vi "Defender_din.vi"(9 "balls":T1[](array[typedef]), 10 "IA State":T2={"our_robots"=[], "enemy_robots"=[], "balls"=[], "geometry"={"field_length"=0, "field_width"=0, "goal_width"=0, "goal_depth"=0, "center_circle_radius"=0, "defense_width"=0, "defense_depth"=0, "free_kick_from_defense_dist"=0, "penalty_spot_from_field_line_dist"=0, "penalty_line_from_spot_dist"=0, "half_moon_depth"=0, "half_moon_width"=0}, "IA Judge"={"stage"="", "command"="", "our_goalie_id"=0.0, "enemy_goalie_id"=0.0, "command enum"=enum."Halt", "Time"=enum."Azul"}, "Received Timestamp"=timestamp(0 s since 1904-01-01), "Events"={"Touch"=FALSE, "id touch"=0.0, "Ball out of \nVision"=FALSE, "Ball inside \nGoalie area"=FALSE, "Robot not responding"=FALSE, "Robots responding status"=[1.0, 1.0, 1.0, 1.0, 1.0, 1.0], "Enemy Ball \nPossession"=FALSE, "Id ini Possession"=0.0, "Ball Possesion"=FALSE, "Id Possesion"=0.0, "Ball at\nour goal side"=FALSE, "Ball at\ntouchline"=FALSE, "Ball at\nenemy goal side"=FALSE}}, 11 "Robot in":T3) -> (3 "Robot out":T3)   [LabVIEW 2018]
uses:
  Core/AI Robot.ctl
  Functions Enum.ctl
  AttackerStates.ctl
  Path Planning/RRT/PathDests.ctl
  Path Planning/RRT/PathDest.ctl
  Core/AI Input.ctl
  Core/AI Ball.ctl
  Core/Field Size.ctl
  Core/AI Judge.ctl
  Command Enum.ctl
  Util/Events/Events.ctl
  <vilib>/Analysis/_algsub.llb/Real Vector Norm.vi
  <vilib>/Analysis/NI_AALPro.lvlib
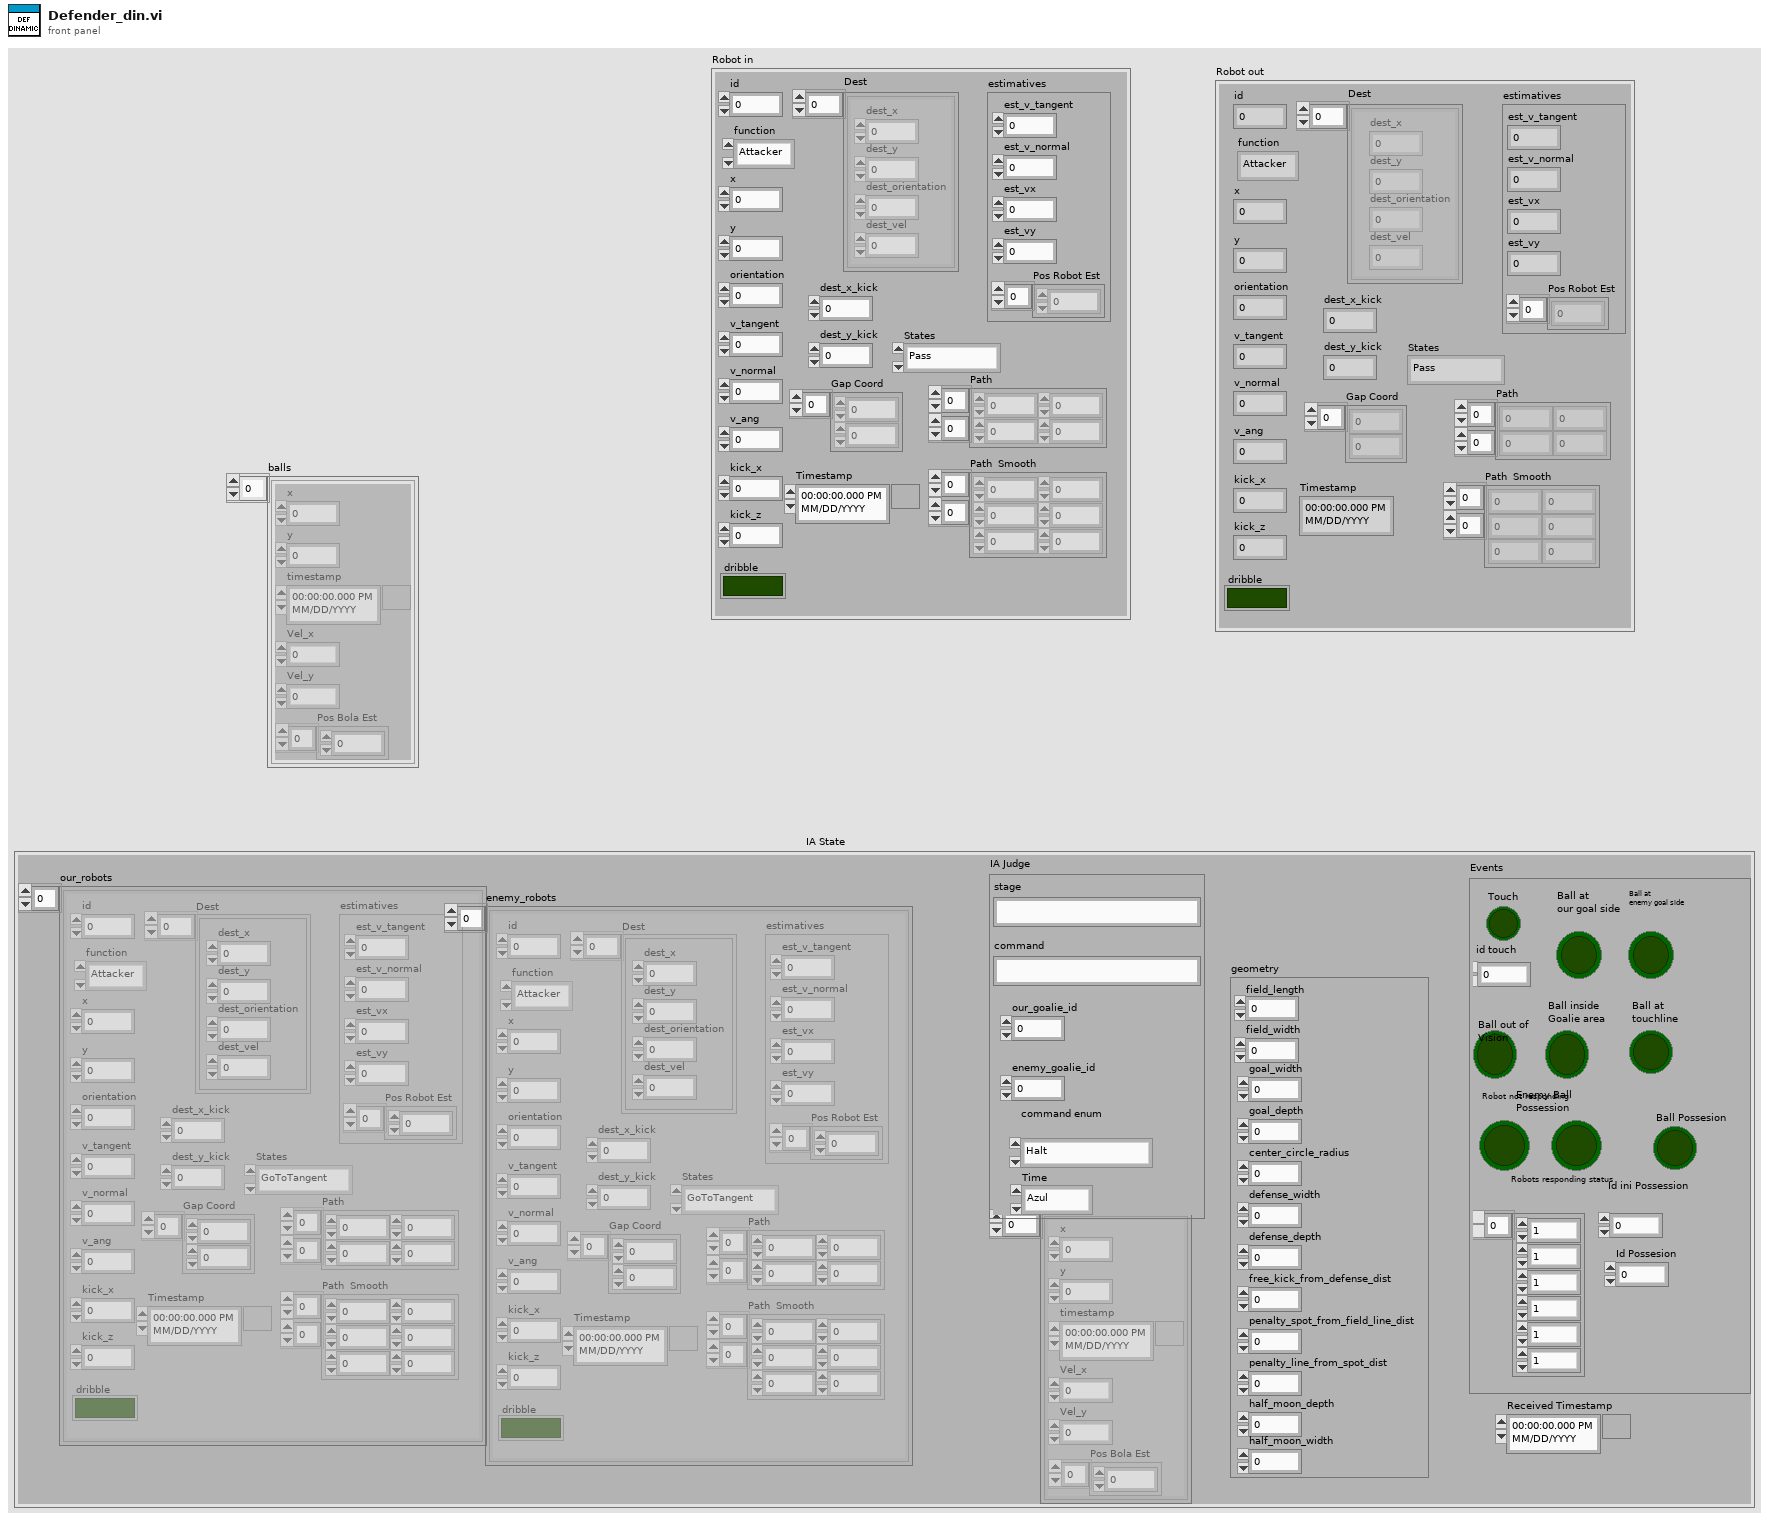
[diagram p1: front panel]
types:
  T1 = typedef "AI Ball.ctl" = cluster{"x":dbl, "y":dbl, "timestamp":timestamp, "Vel_x":dbl, "Vel_y":dbl, "Pos Bola Est":dbl[]}
  T2 = typedef "AI Input.ctl" = cluster{"our_robots":T3[], "enemy_robots":T3[], "balls":T1[], "geometry":T8, "IA Judge":T9, "Received Timestamp":timestamp, "Events":T11}
  T3 = typedef "AI Robot.ctl" = cluster{"id":u32, "function":T4, "x":dbl, "y":dbl, "orientation":dbl, "v_tangent":dbl, "v_normal":dbl, "v_ang":dbl, "kick_x":dbl, "kick_z":dbl, "dribble":bool, "Timestamp":timestamp, "estimatives":cluster{"est_v_tangent":dbl, "est_v_normal":dbl, "est_vx":dbl, "est_vy":dbl, "Pos Robot Est":dbl[]}, "dest_x_kick":dbl, "dest_y_kick":dbl, "Gap Coord":dbl[], "States":T5, "Path ":dbl[][], "Path  Smooth":dbl[][], "Dest":T6}
  T4 = typedef "Functions Enum.ctl" = enum16{"Attacker", "Goalie", "Defender", "Striker", "Goto 0", "Dummy", "Kicker", "ZigZag"}
  T5 = typedef "AttackerStates.ctl" = enum16{"Pass", "GoToTangent", "BallGetting", "GoToKick", "Rotate anti-clockwise", "Rotate Clockwise", ""}
  T6 = typedef "PathDests.ctl" = T7[]
  T7 = typedef "PathDest.ctl" = cluster{"dest_x":dbl, "dest_y":dbl, "dest_orientation":dbl, "dest_vel":dbl}
  T8 = typedef "Field Size.ctl" = cluster{"field_length":u32, "field_width":u32, "goal_width":u32, "goal_depth":u32, "center_circle_radius":u32, "defense_width":u32, "defense_depth":u32, "free_kick_from_defense_dist":u32, "penalty_spot_from_field_line_dist":u32, "penalty_line_from_spot_dist":u32, "half_moon_depth":u32, "half_moon_width":u32}
  T9 = typedef "AI Judge.ctl" = cluster{"stage":string, "command":string, "our_goalie_id":dbl, "enemy_goalie_id":dbl, "command enum":T10, "Time":enum16{"Azul", "Amarelo"}}
  T10 = typedef "Command Enum.ctl" = enum16{"Halt", "Stop", "Force Start", "PKA Normal Start", "Prepare Kickoff Ally", "PKE Normal Start", "Prepare Kickoff Enemy", "Prepare Penalty Ally", "PPA Normal Start", "Prepare Penalty Enemy", "PPE Normal Start", "Ball Placement Enemy Up", "Ball Placement Enemy Down", "Ball Placement Ally Up", "Ball Placement Ally Mid", "Ball Placement Ally Down", "Indirect Free Enemy", "Indirect Free Ally", "Timeout Enemy", "Timeout Ally", "Goal Enemy", "Goal Ally", "Normal Half Time", "Extra Time Break", "Extra Half Time", "None", "Post Game"}
  T11 = typedef "Events.ctl" = cluster{"Touch":bool, "id touch":dbl, "Ball out of \nVision":bool, "Ball inside \nGoalie area":bool, "Robot not responding":bool, "Robots responding status":dbl[], "Enemy Ball \nPossession":bool, "Id ini Possession":dbl, "Ball Possesion":bool, "Id Possesion":dbl, "Ball at\nour goal side":bool, "Ball at\ntouchline":bool, "Ball at\nenemy goal side":bool}
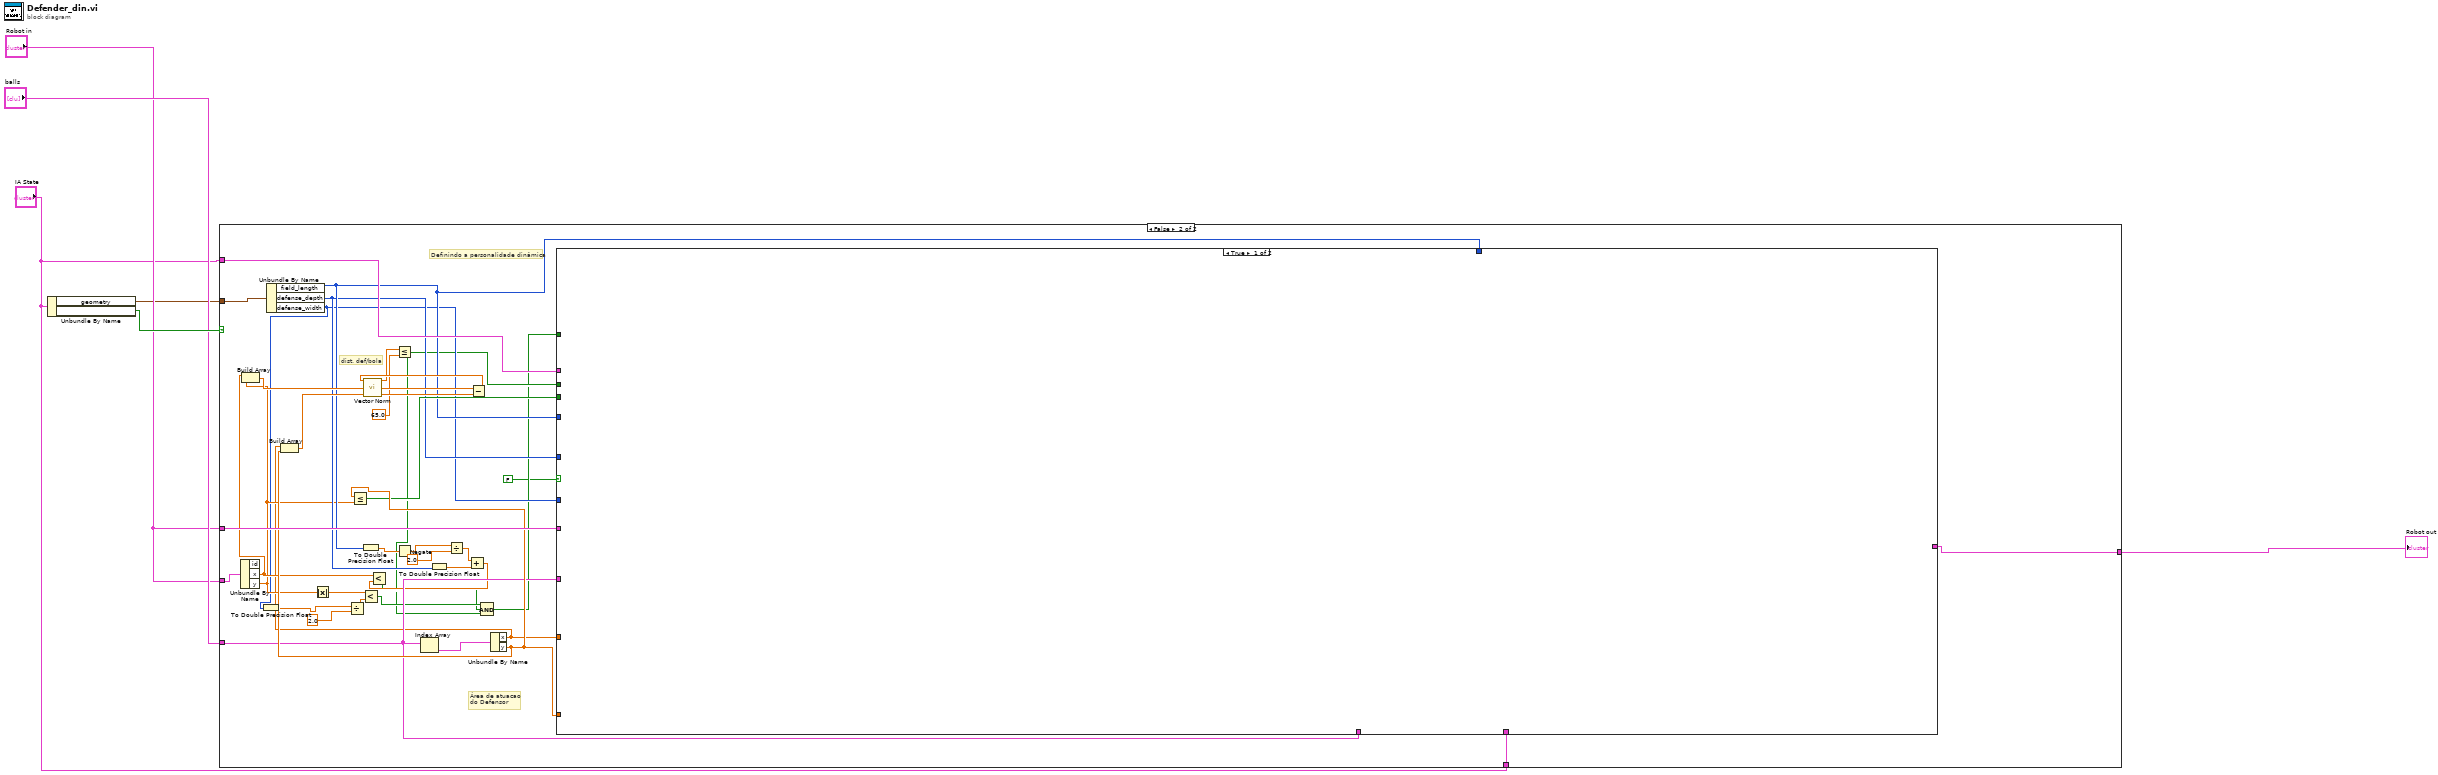
[diagram p0: block diagram]
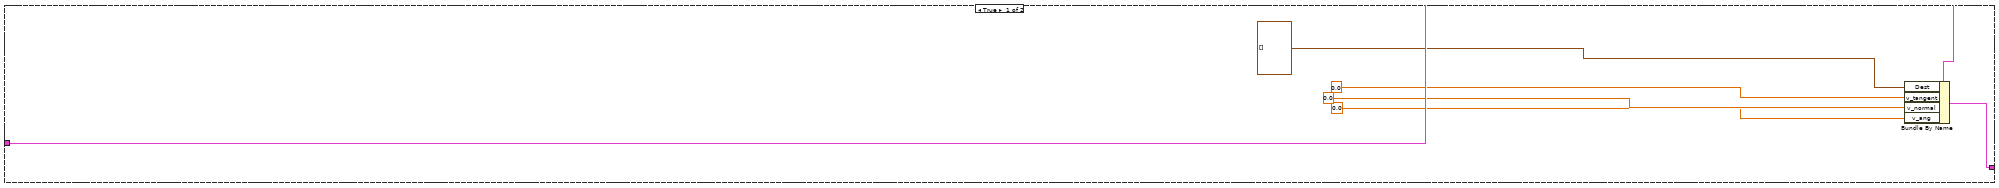
[diagram p2: hidden frame]
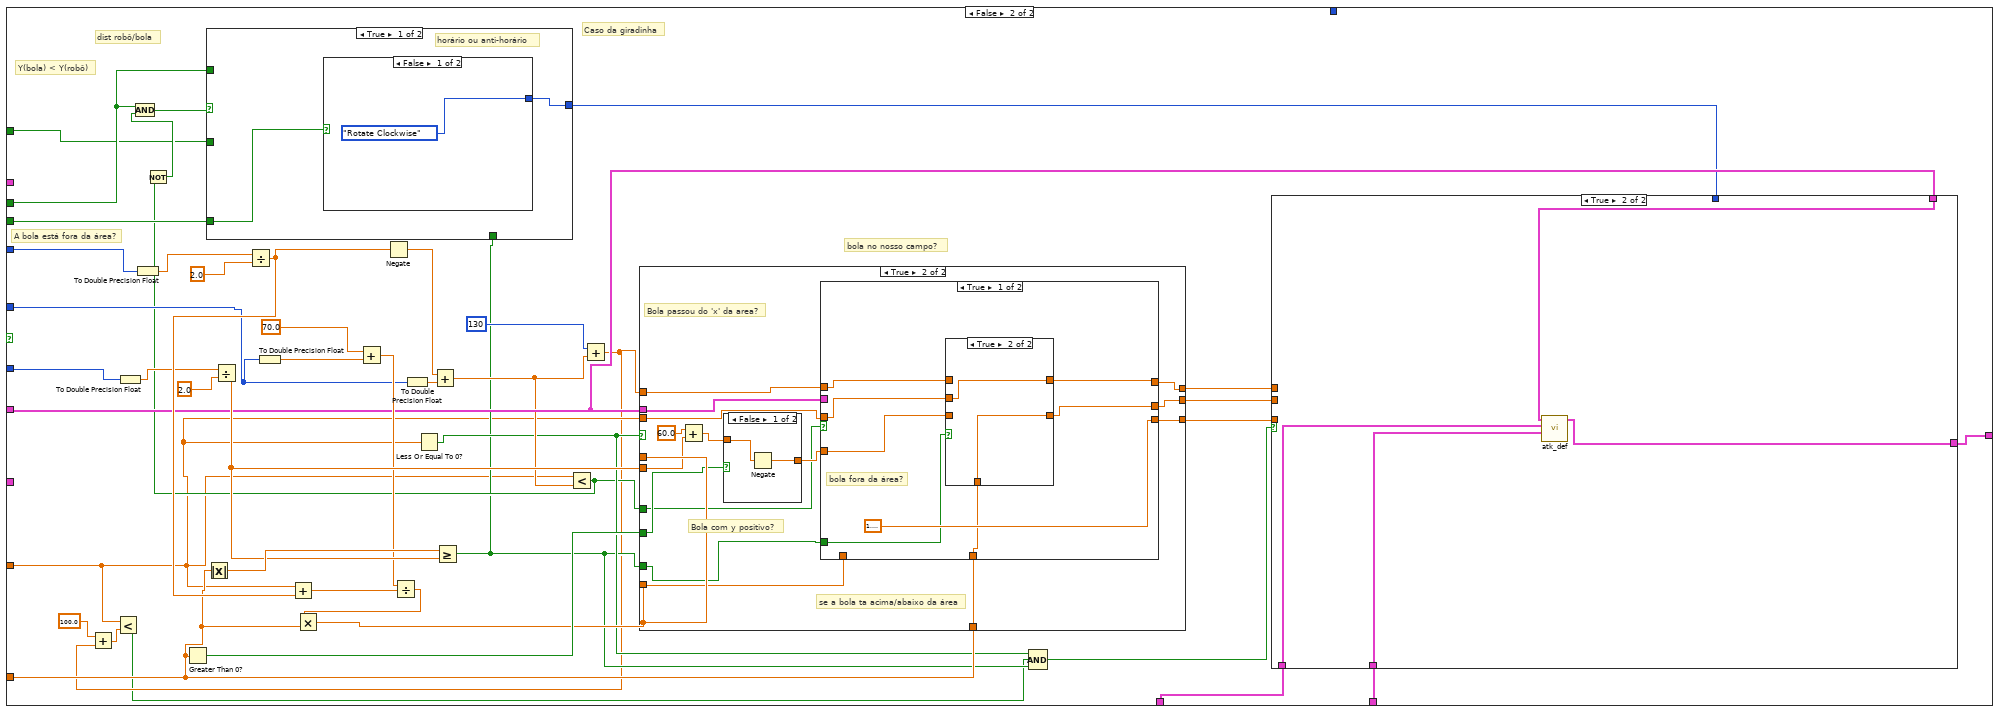
[diagram p3: hidden frame]
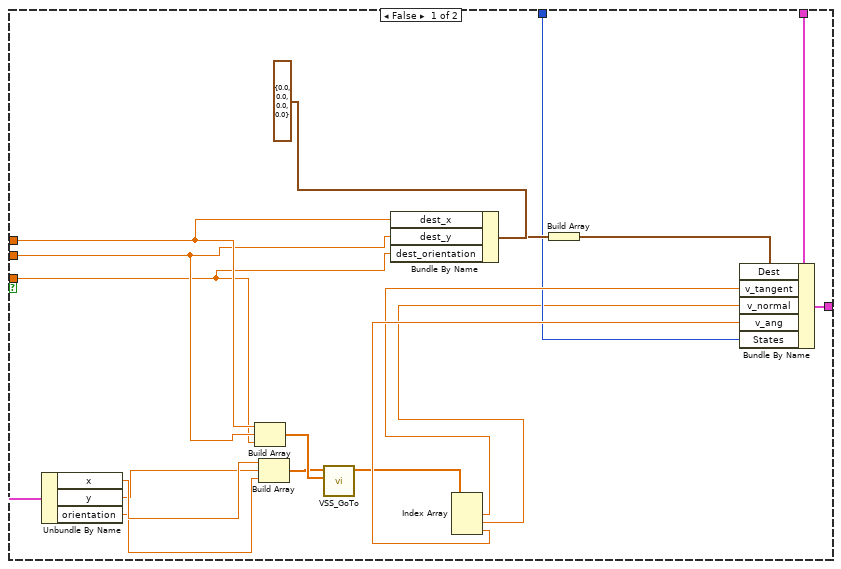
[diagram p4: hidden frame]
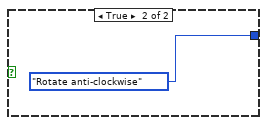
[diagram p5: hidden frame]
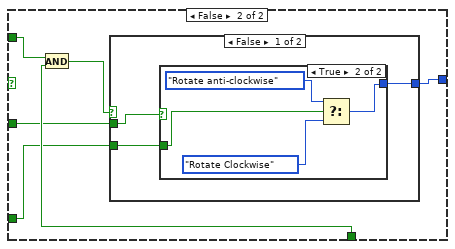
[diagram p6: hidden frame]
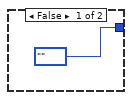
[diagram p7: hidden frame]
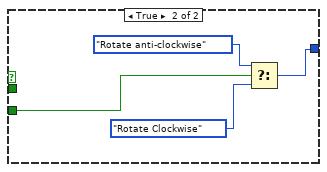
[diagram p8: hidden frame]
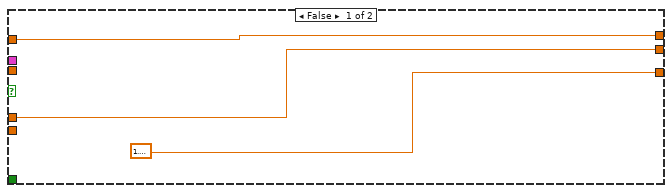
[diagram p9: hidden frame]
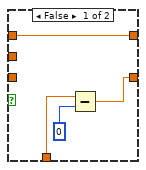
[diagram p11: hidden frame]
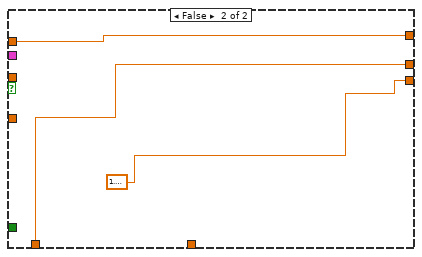
[diagram p12: hidden frame]
diagram:
  n1 = Unbundle By Name("IA State") -> ("geometry"=w3:T8, "Events.Ball out of \nVision"=w6:bool)
  n2 = case shown="False" w6 {
    tunnel: "Robot in" -> [w11 w48]
    tunnel: "balls" -> [_ w35]
    tunnel: "Robot in" -> [_ w46]
    tunnel: w3 -> [_ w45]
    tunnel: "IA State" -> [_ w44]
    tunnel: [w12 w43] -> w2
    tunnel: "IA State" -> [_ w34]
    frame True {
      n3 = Bundle By Name(cluster=w11, "Dest"=T7[] [], "v_tangent"=0.0, "v_normal"=0.0, "v_ang"=0.0) -> (w12:T3)
    }
    frame False {
      # "Área de atuacao\ndo Defensor"
      # "dist. def/bola"
      # "Definindo a personalidade dinâmica"
      n4 = Unbundle By Name(w46) -> ("x"=w33:dbl, "y"=w24:dbl)  [unwired: 1 out]
      n5 = Build Array(w33, w24) -> (w42:dbl[])
      n6 = Unbundle By Name(w45) -> ("field_length"=w29:u32, "defense_depth"=w27:u32, "defense_width"=w21:u32)
      n7 = To Double Precision Float(number=w21) -> (double precision float=w15:dbl)
      n8 = Absolute Value(x=w24) -> (abs(x)=w23:dbl)
      n9 = Divide(x=w15, y=2.0) -> (x/y=w20:dbl)
      n10 = To Double Precision Float(number=w29) -> (double precision float=w30:dbl)
      n11 = Less?(x=w23, y=w20) -> (x < y?=w19:bool)
      n12 = Negate(x=w30) -> (-x=w31:dbl)
      n13 = Index Array(array=w35) -> (element=w47:T1)  [unwired: 1 in]
      n14 = To Double Precision Float(number=w27) -> (double precision float=w26:dbl)
      n15 = Divide(x=w31, y=2.0) -> (x/y=w28:dbl)
      n16 = Add(x=w28, y=w26) -> (x+y=w25:dbl)
      n17 = Less?(x=w33, y=w25) -> (x < y?=w18:bool)
      n18 = Unbundle By Name(w47) -> ("x"=w14:dbl, "y"=w37:dbl)
      n19 = Build Array(w14, w37) -> (w41:dbl[])
      n20 = Less Or Equal?(x=w37, y=w24) -> (x <= y?=w36:bool)
      n21 = Subtract(x=w42, y=w41) -> (x-y=w40:dbl[])
      n22 = call-poly <vilib>:"Vector Norm.vi"("Input Vector"=w40) -> ("norm"=w39:dbl)  [unwired: 9 in, 1 out]
      n23 = Less Or Equal?(x=w39, y=65.0) -> (x <= y?=w17:bool)
      n24 = Compound Arithmetic op=AND(w19, w18, w17) -> (w16:bool)
      n25 = case shown="True" FALSE {
        tunnel: w48 -> [_ w75]
        tunnel: w14 -> [_ w53]
        tunnel: w37 -> [_ w79]
        tunnel: w29 -> [_ w73]
        tunnel: w27 -> [_ w70]
        tunnel: w21 -> [_ w67]
        tunnel: w44 -> [_ _]
        tunnel: w35 -> [_ _]
        tunnel: [_ w74] -> w43
        tunnel: w17 -> [_ w61]
        tunnel: w36 -> [_ w64]
        tunnel: w35 -> [_ w56]
        tunnel: w29 -> [_ _]
        tunnel: w34 -> [_ w55]
        tunnel: w16 -> [_ w54]
        frame True {
        }
        frame False {
          # "Y(bola) < Y(robô)"
          # "dist robô/bola"
          # "A bola está fora da área?"
          # "Caso da giradinha"
          # "bola no nosso campo?"
          n26 = To Double Precision Float(number=w67) -> (double precision float=w66:dbl)
          n27 = To Double Precision Float(number=w73) -> (double precision float=w72:dbl)
          n28 = Greater Than 0?(x=w79) -> (x > 0?=w86:bool)
          n29 = Absolute Value(x=w79) -> (abs(x)=w91:dbl)
          n30 = Divide(x=w66, y=2.0) -> (x/y=w83:dbl)
          n31 = Divide(x=w72, y=2.0) -> (x/y=w85:dbl)
          n32 = To Double Precision Float(number=w70) -> (double precision float=w71:dbl)
          n33 = Add(x=w53, y=w85) -> (x+y=w84:dbl)
          n34 = Add(x=70.0, y=w71) -> (x+y=w81:dbl)
          n35 = Negate(x=w85) -> (-x=w90:dbl)
          n36 = Divide(x=w81, y=w84) -> (x/y=w88:dbl)
          n37 = Multiply(x=w88, y=w79) -> (x*y=w80:dbl)
          n38 = To Double Precision Float(number=w70) -> (double precision float=w69:dbl)
          n39 = Less Or Equal To 0?(x=w53) -> (x <= 0?=w60:bool)
          n40 = Add(x=w90, y=w69) -> (x+y=w62:dbl)
          n41 = Greater Or Equal?(x=w91, y=w83) -> (x >= y?=w58:bool)
          n42 = Less?(x=w53, y=w62) -> (x < y?=w59:bool)
          n43 = Not(x=w59) -> (.not. x?=w63:bool)
          n44 = Compound Arithmetic op=AND(w61, w63) -> (w65:bool)
          n45 = case shown="True" w65 {
            tunnel: [w115 w124] -> w68
            tunnel: w64 -> [w116 w120]
            tunnel: w61 -> [_ w123]
            tunnel: w58 -> [_ w122]
            tunnel: w54 -> [_ w119]
            frame True {
              # "horário ou anti-horário"
              n46 = case shown="False" w116 {
                tunnel: [AttackerStates."Rotate Clockwise" ("States") AttackerStates."Rotate anti-clockwise" ("States")] -> w115
                frame False {
                }
                frame True {
                }
              }
            }
            frame False {
              n47 = And(x=w123, y=w122) -> (x .and. y?=w121:bool)
              n48 = case shown="False" w121 {
                tunnel: [w127 w135] -> w124
                tunnel: w120 -> [w125 w136]
                tunnel: w119 -> [w126 _]
                frame False {
                  n49 = case shown="True" w126 {
                    tunnel: [AttackerStates."" ("States") w129] -> w127
                    tunnel: w125 -> [_ w130]
                    frame False {
                    }
                    frame True {
                      n50 = Select(t=AttackerStates."Rotate anti-clockwise" ("States"), s=w130, f=AttackerStates."Rotate Clockwise" ("States")) -> (s? t:f=w129:T5)
                    }
                  }
                }
                frame True {
                  n51 = Select(t=AttackerStates."Rotate anti-clockwise" ("States"), s=w136, f=AttackerStates."Rotate Clockwise" ("States")) -> (s? t:f=w135:T5)
                }
              }
            }
          }
          n52 = Add(x=130, y=w62) -> (x+y=w51:dbl)
          n53 = Add(x=100.0, y=w51) -> (x+y=w52:dbl)
          n54 = Less?(x=w53, y=w52) -> (x < y?=w49:bool)
          n55 = case shown="True" w60 {
            tunnel: w75 -> [_ w154]
            tunnel: w51 -> [w139 w153]
            tunnel: w59 -> [_ w140]
            tunnel: w86 -> [_ w152]
            tunnel: w83 -> [_ w145]
            tunnel: w53 -> [_ w151]
            tunnel: w80 -> [w138 _]
            tunnel: w58 -> [_ w143]
            tunnel: [w139 w150] -> w78
            tunnel: [w138 w149] -> w77
            tunnel: [1.5707963267948966 w148] -> w76
            tunnel: w79 -> [_ w144]
            tunnel: w80 -> [_ w141]
            frame False {
            }
            frame True {
              # "se a bola ta acima/abaixo da área"
              # "Bola passou do 'x' da area?"
              # "Bola com y positivo?"
              n56 = Add(x=60.0, y=w145) -> (x+y=w147:dbl)
              n57 = case shown="False" w152 {
                tunnel: w147 -> [w156 w157]
                tunnel: [w155 w157] -> w142
                frame False {
                  n58 = Negate(x=w156) -> (-x=w155:dbl)
                }
                frame True {
                }
              }
              n59 = case shown="True" w140 {
                tunnel: w154 -> [_ _]
                tunnel: w142 -> [w162 _]
                tunnel: w153 -> [w161 w174]
                tunnel: w151 -> [w159 _]
                tunnel: [w160 w174] -> w150
                tunnel: [w164 w172] -> w149
                tunnel: [1.5707963267948966 1.5707963267948966] -> w148
                tunnel: w143 -> [w158 _]
                tunnel: w144 -> [w163 _]
                tunnel: w141 -> [_ w172]
                frame True {
                  # "bola fora da área?"
                  n60 = case shown="True" w158 {
                    tunnel: w162 -> [_ _]
                    tunnel: [w166 w170] -> w164
                    tunnel: w163 -> [w168 w170]
                    tunnel: w161 -> [w169 _]
                    tunnel: [w169 w171] -> w160
                    tunnel: w159 -> [_ w171]
                    frame False {
                      n61 = Subtract(x=w168, y=0) -> (x-y=w166:dbl)
                    }
                    frame True {
                    }
                  }
                }
                frame False {
                }
              }
            }
          }
          n62 = Compound Arithmetic op=AND(w60, w49, w58) -> (w57:bool)
          n63 = case shown="True" w57 {
            tunnel: w78 -> [w102 _]
            tunnel: w77 -> [w101 _]
            tunnel: w76 -> [w100 _]
            tunnel: w75 -> [w99 w113]
            tunnel: [w98 w114] -> w74
            tunnel: w68 -> [w97 _]
            tunnel: w56 -> [_ w112]
            tunnel: w55 -> [_ w111]
            frame False {
              n64 = Unbundle By Name(w99) -> ("x"=w105:dbl, "y"=w103:dbl, "orientation"=w104:dbl)
              n65 = Build Array(w102, w101, w100) -> (w94:dbl[])
              n66 = Build Array(w105, w103, w104) -> (w93:dbl[])
              n67 = call "VSS_GoTo.vi"("SetPoint"=w94, "Position"=w93) -> ("Output Vel"=w95:dbl[])  [unwired: 9 in]
              n68 = Bundle By Name(cluster=T7 {"dest_x"=0.0, "dest_y"=0.0, "dest_orientation"=0.0, "dest_vel"=0.0} ("element"), "dest_x"=w102, "dest_y"=w101, "dest_orientation"=w100) -> (w106:T7)
              n69 = Index Array(array=w95) -> (element #1=w109:dbl, element #2=w96:dbl, element #3=w110:dbl)  [unwired: 3 in]
              n70 = Build Array(w106) -> (w108:T7[])
              n71 = Bundle By Name(cluster=w99, "Dest"=w108, "v_tangent"=w109, "v_normal"=w96, "v_ang"=w110, "States"=w97) -> (w98:T3)
            }
            frame True {
              n72 = call "atk_def.vi"("IA State"=w111, "balls"=w112, "Robot in"=w113) -> ("Robot out"=w114:T3)  [unwired: 8 in]
            }
          }
        }
      }
    }
  }
  "Robot out" <- w2
